vi "Get API.vi"(8 "error in (no error)":errorcluster, 11 "Test 1 in":refnum<class "Test 1.lvclass">) -> (0 "error out":errorcluster, 2 "Actor API":refnum<class "Actor API.lvclass">, 3 "Test 1 out":refnum<class "Test 1.lvclass">)   [LabVIEW 2020, in "Scratchpad.lvlib" / "Test 1.lvlib" / "Test 1.lvclass"]
uses:
  Test 1.lvclass
  Artifex/Actor Proxy/Actor API.lvclass
  Test 1.lvclass/Test 1.ctl
  Test 1 API/Test 1 API.lvclass
  C:/dev/lv20CE/relink/lv-artifex/Artifex/Actor Proxy/Actor API.lvclass
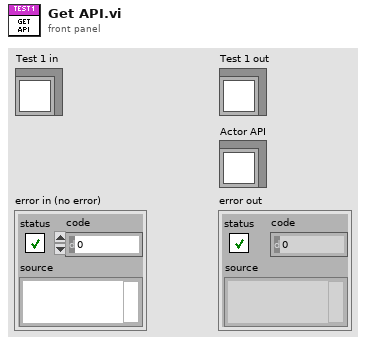
[diagram p1: front panel]
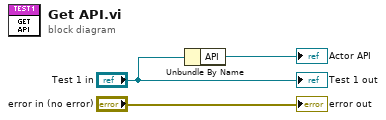
[diagram p0: block diagram]
diagram:
  n1 = Unbundle By Name("Test 1 in") -> ("API"=→"Actor API":refnum<class "Test 1 API.lvclass">)
  "error out" <- "error in (no error)"
  "Test 1 out" <- "Test 1 in"
